vi "Set Active.vi"(10 "active":bool, 11 "Plugin in":refnum<class "Plugin.lvclass">) -> (3 "Plugin out":refnum<class "Plugin.lvclass">)   [LabVIEW 2021, in "DSF Core.lvlib" / "Plugin.lvclass"]
uses:
  Plugin.lvclass
  Plugin.lvclass/Plugin.ctl
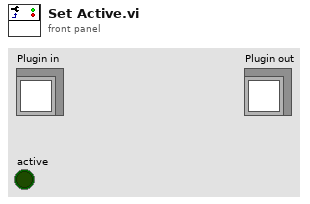
[diagram p1: front panel]
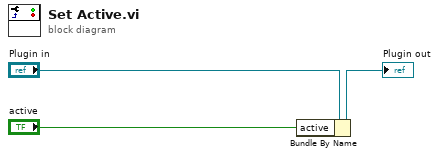
[diagram p0: block diagram]
diagram:
  n1 = Bundle By Name(cluster="Plugin in", "active"="active") -> (→"Plugin out":refnum<class "Plugin.lvclass">)
